vi "ReadDashValues.vi"(8 "error in (no error)":errorcluster) -> (0 "error out":errorcluster, 2 "output cluster":T1)   [LabVIEW 2014]
uses:
  buttons/PresetValues.ctl
  <vilib>/Utility/config.llb/Read Key (Double).vi
  <vilib>/Utility/config.llb/NI_LVConfig.lvlib
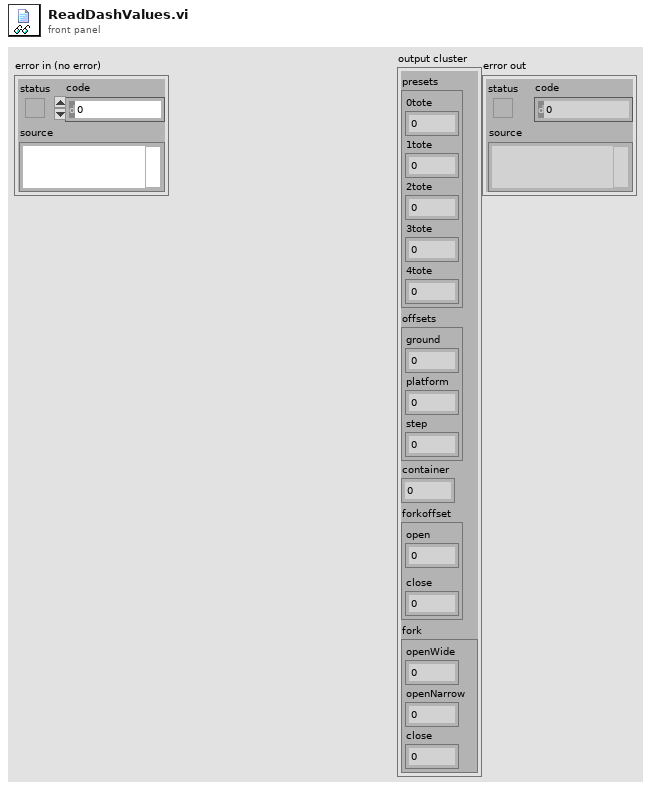
[diagram p1: front panel]
types:
  T1 = typedef "PresetValues.ctl" = cluster{"presets":cluster{"0tote":dbl, "1tote":dbl, "2tote":dbl, "3tote":dbl, "4tote":dbl}, "offsets":cluster{"ground":dbl, "platform":dbl, "step":dbl}, "container":dbl, "forkoffset":cluster{"open":dbl, "close":dbl}, "fork":cluster{"openWide":dbl, "openNarrow":dbl, "close":dbl}}
  T2 = typedef "NI_LVConfig.lvlib/Config Data RefNum.ctl" = refnum<k1>
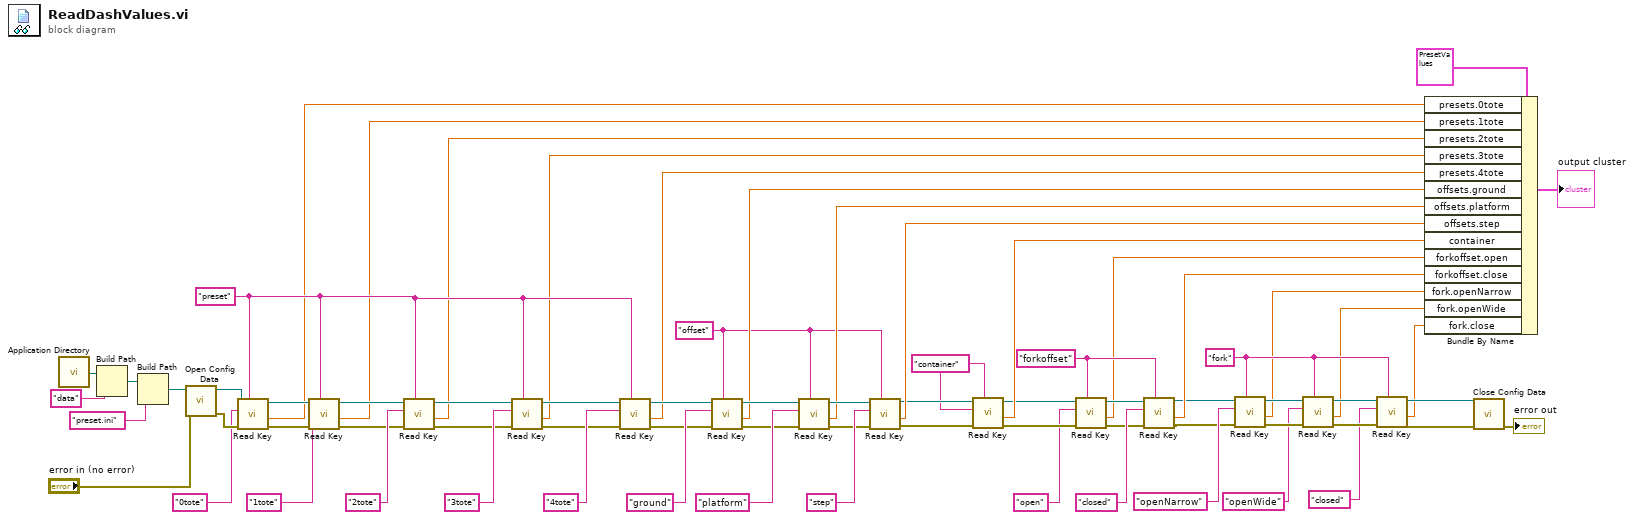
[diagram p0: block diagram]
diagram:
  w10 = "fork" ("section")
  w20 = "forkoffset" ("section")
  w29 = "container" ("section")
  w38 = "offset" ("section")
  w50 = "preset" ("section")
  n1 = call <vilib>:"Application Directory.vi"() -> ("Application Directory"=w68:path)
  n2 = Build Path(base path=w68, name or relative path="data") -> (appended path=w66:path)
  n3 = Build Path(base path=w66, name or relative path="preset.ini") -> (appended path=w64:path)
  n4 = call <vilib>:"Open Config Data.vi"("error in (no error)"="error in (no error)", "configuration file path"=w64) -> ("error out"=w71:errorcluster, "refnum"=w70:T2)  [unwired: 7 in, 1 out]
  n5 = call-poly <vilib>:"Read Key.vi"("section"=w50, "error in (no error)"=w71, "key"="0tote", "refnum"=w70) -> ("error out"=w36:errorcluster, "value"=w46:dbl, "refnum out"=w63:T2)  [unwired: 4 in, 1 out]
  n6 = call-poly <vilib>:"Read Key.vi"("section"=w50, "error in (no error)"=w36, "key"="1tote", "refnum"=w63) -> ("error out"=w35:errorcluster, "value"=w47:dbl, "refnum out"=w61:T2)  [unwired: 4 in, 1 out]
  n7 = call-poly <vilib>:"Read Key.vi"("section"=w50, "error in (no error)"=w35, "key"="2tote", "refnum"=w61) -> ("error out"=w34:errorcluster, "value"=w45:dbl, "refnum out"=w59:T2)  [unwired: 4 in, 1 out]
  n8 = call-poly <vilib>:"Read Key.vi"("section"=w50, "error in (no error)"=w34, "key"="3tote", "refnum"=w59) -> ("error out"=w33:errorcluster, "value"=w44:dbl, "refnum out"=w57:T2)  [unwired: 4 in, 1 out]
  n9 = call-poly <vilib>:"Read Key.vi"("section"=w50, "error in (no error)"=w33, "key"="4tote", "refnum"=w57) -> ("error out"=w32:errorcluster, "value"=w43:dbl, "refnum out"=w55:T2)  [unwired: 4 in, 1 out]
  n10 = call-poly <vilib>:"Read Key.vi"("section"=w38, "error in (no error)"=w32, "key"="ground", "refnum"=w55) -> ("error out"=w31:errorcluster, "value"=w42:dbl, "refnum out"=w54:T2)  [unwired: 4 in, 1 out]
  n11 = call-poly <vilib>:"Read Key.vi"("section"=w38, "error in (no error)"=w31, "key"="platform", "refnum"=w54) -> ("error out"=w30:errorcluster, "value"=w41:dbl, "refnum out"=w51:T2)  [unwired: 4 in, 1 out]
  n12 = call-poly <vilib>:"Read Key.vi"("section"=w38, "error in (no error)"=w30, "key"="step", "refnum"=w51) -> ("error out"=w27:errorcluster, "value"=w40:dbl, "refnum out"=w37:T2)  [unwired: 4 in, 1 out]
  n13 = call-poly <vilib>:"Read Key.vi"("section"=w29, "error in (no error)"=w27, "key"=w29, "refnum"=w37) -> ("error out"=w25:errorcluster, "value"=w28:dbl, "refnum out"=w26:T2)  [unwired: 4 in, 1 out]
  n14 = call-poly <vilib>:"Read Key.vi"("section"=w20, "error in (no error)"=w25, "key"="open", "refnum"=w26) -> ("error out"=w23:errorcluster, "value"=w19:dbl, "refnum out"=w22:T2)  [unwired: 4 in, 1 out]
  n15 = call-poly <vilib>:"Read Key.vi"("section"=w20, "error in (no error)"=w23, "key"="closed", "refnum"=w22) -> ("error out"=w12:errorcluster, "value"=w18:dbl, "refnum out"=w13:T2)  [unwired: 4 in, 1 out]
  n16 = call-poly <vilib>:"Read Key.vi"("section"=w10, "error in (no error)"=w12, "key"="openNarrow", "refnum"=w13) -> ("error out"=w15:errorcluster, "value"=w5:dbl, "refnum out"=w16:T2)  [unwired: 4 in, 1 out]
  n17 = call-poly <vilib>:"Read Key.vi"("section"=w10, "error in (no error)"=w15, "key"="openWide", "refnum"=w16) -> ("error out"=w7:errorcluster, "value"=w4:dbl, "refnum out"=w11:T2)  [unwired: 4 in, 1 out]
  n18 = call-poly <vilib>:"Read Key.vi"("section"=w10, "error in (no error)"=w7, "key"="closed", "refnum"=w11) -> ("error out"=w8:errorcluster, "value"=w3:dbl, "refnum out"=w9:T2)  [unwired: 4 in, 1 out]
  n19 = Bundle By Name(cluster=T1 {"presets"={"0tote"=0.0, "1tote"=0.0, "2tote"=0.0, "3tote"=0.0, "4tote"=0.0}, "offsets"={"ground"=0.0, "platform"=0.0, "step"=0.0}, "container"=0.0, "forkoffset"={"open"=0.0, "close"=0.0}, "fork"={"openWide"=0.0, "openNarrow"=0.0, "close"=0.0}}, "presets.0tote"=w46, "presets.1tote"=w47, "presets.2tote"=w45, "presets.3tote"=w44, "presets.4tote"=w43, "offsets.ground"=w42, "offsets.platform"=w41, "offsets.step"=w40, "container"=w28, "forkoffset.open"=w19, "forkoffset.close"=w18, "fork.openNarrow"=w5, "fork.openWide"=w4, "fork.close"=w3) -> (→"output cluster":T1)
  n20 = call <vilib>:"Close Config Data.vi"("error in (no error)"=w8, "refnum"=w9) -> ("error out"=→"error out":errorcluster)  [unwired: 8 in, 1 out]
